vi "Histogram.vi"(0 "image in":refnum<class "MSC Image.lvclass">, 5 "error in (no error)":errorcluster) -> (14 "image out":refnum<class "MSC Image.lvclass">, 15 "R":T1, 16 "G":T1, 17 "B":T1, 19 "error out":errorcluster)   [LabVIEW 2014, in "MSC Image.lvclass"]
doc: "Calculates the histogram of the image. You can wire the outputs directly to a XY Graph.\n\nThe image type double can lead to overflows."
uses:
  MSC Image.lvclass
  <vilib>/Analysis/NI_AALPro.lvlib
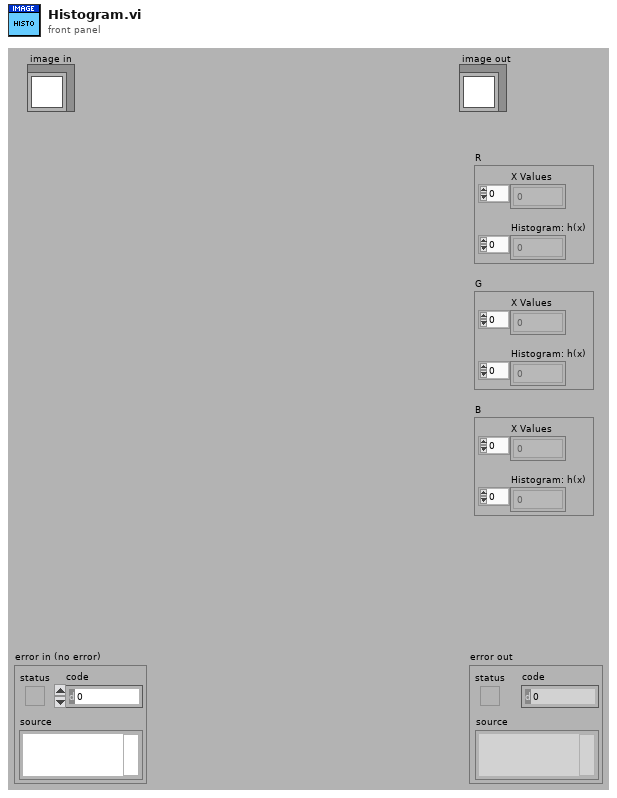
[diagram p1: front panel]
types:
  T1 = cluster{"X Values":dbl[], "Histogram: h(x)":dbl[]}
  T2 = typedef "MSC Image.lvclass/Image Type.ctl" = i32
  T3 = cluster{"X Values":dbl[], "Histogram: h(x)":i32[]}
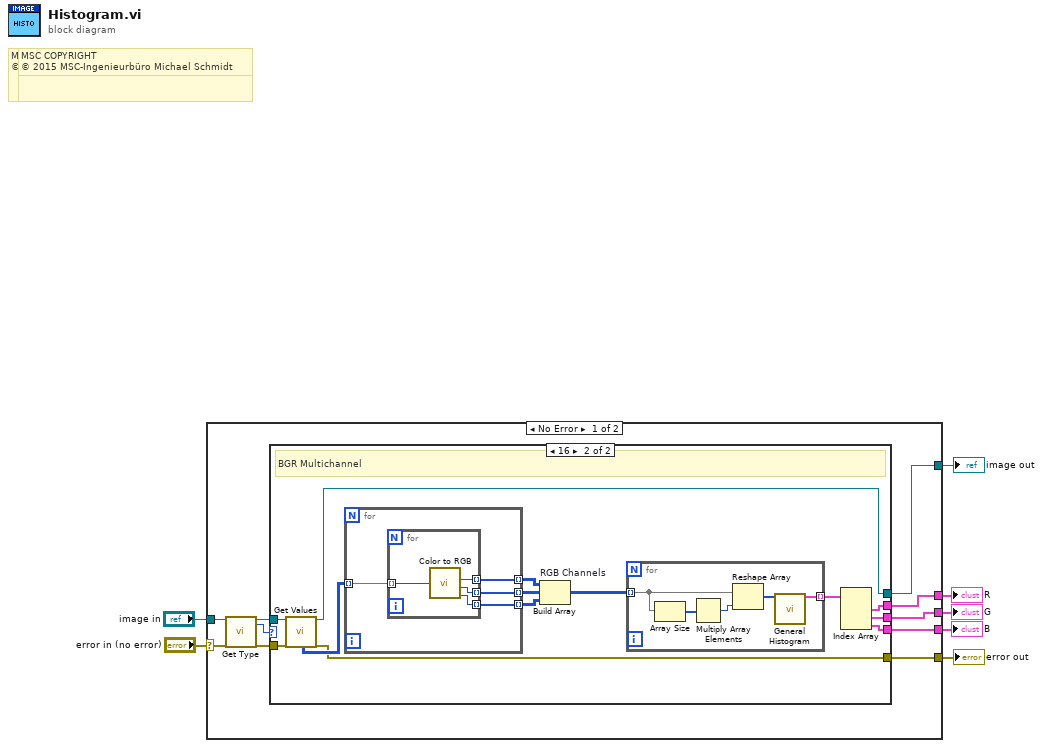
[diagram p0: block diagram]
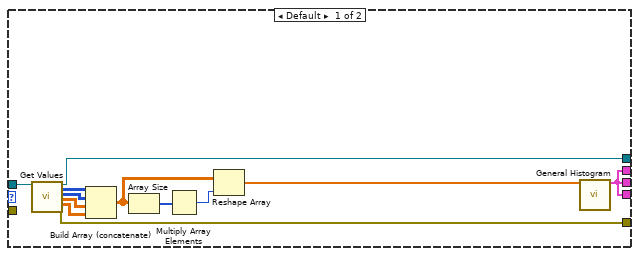
[diagram p2: hidden frame]
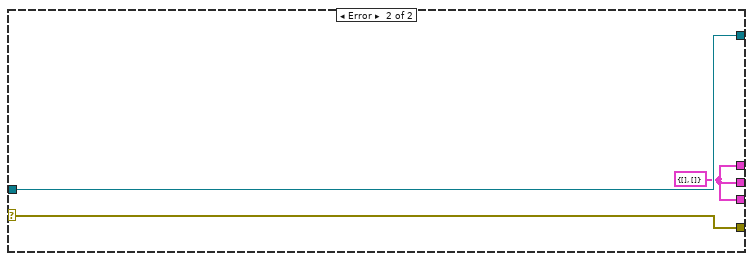
[diagram p3: hidden frame]
diagram:
  # "MSC COPYRIGHT\n© 2016 MSC-Ingenieurbüro Michael Schmidt"
  # "MSC COPYRIGHT\n© 2016 MSC-Ingenieurbüro Michael Schmidt"
  # "MSC COPYRIGHT\n© 2015 MSC-Ingenieurbüro Michael Schmidt"
  # "MSC COPYRIGHT\n© 2015 MSC-Ingenieurbüro Michael Schmidt"
  n1 = case shown="No Error" "error in (no error)" {
    selector: "error in (no error)" -> [w12 w58]
    tunnel: [w13 w58] -> w5
    tunnel: [w17 w57] -> w6
    tunnel: "image in" -> [w10 w57]
    tunnel: [w16 w56] -> w3
    tunnel: [w15 w56] -> w2
    tunnel: [w14 w56] -> w1
    frame No Error {
      n2 = call-dynamic "Get Type.vi"("image in"=w10, "error in (no error)"=w12) -> ("image out"=w9:refnum<class "MSC Image.lvclass">, "Image Type"=w8:T2, "error out"=w11:errorcluster)  [unwired: 15 in]
      n3 = case shown="16" w8 {
        tunnel: w9 -> [w24 w34]
        tunnel: [w23 w32] -> w17
        tunnel: [w29 w37] -> w16
        tunnel: [w29 w36] -> w15
        tunnel: [w29 w35] -> w14
        tunnel: w11 -> [_ w33]
        tunnel: [w18 w30] -> w13
        frame Default {
          n4 = call-dynamic "Get Values.vi"("image in"=w24) -> ("image out"=w23:refnum<class "MSC Image.lvclass">, "imageData U8"=w22:u8[][], "imageData U16"=w21:u16[][], "imageData Single"=w20:sgl[][], "imageData Double"=w19:dbl[][], "error out"=w18:errorcluster)  [unwired: 11 in, 2 out]
          n5 = Build Array (concatenate)(w22, w21, w20, w19) -> (w26:dbl[][])
          n6 = Array Size(array=w26) -> (size(s)=w27:i32[])
          n7 = Multiply Array Elements(1:w27) -> (0:w28:i32)
          n8 = Reshape Array(w26, w28) -> (w25:dbl[])
          n9 = call <vilib>:"General Histogram.vi"("X"=w25) -> ("Histogram Graph"=w29:T3)  [unwired: 10 in, 4 out]
        }
        frame 16 {
          # "BGR Multichannel"
          n10 = call-dynamic "Get Values.vi"("image in"=w34, "error in (no error)"=w33) -> ("imageData BGR"=w31:u32[][], "image out"=w32:refnum<class "MSC Image.lvclass">, "error out"=w30:errorcluster)  [unwired: 10 in, 5 out]
          n11 = for {
            tunnel: w31 -> [w51] mode=indexing
            tunnel: [w50] -> w42 mode=indexing
            tunnel: [w49] -> w41 mode=indexing
            tunnel: [w48] -> w40 mode=indexing
            n12 = for {
              tunnel: w51 -> [w55] mode=indexing
              tunnel: [w54] -> w50 mode=indexing
              tunnel: [w53] -> w49 mode=indexing
              tunnel: [w52] -> w48 mode=indexing
              n13 = call <vilib>:"Color to RGB.vi"("Color"=w55) -> ("R"=w54:u8, "G"=w53:u8, "B"=w52:u8)  [unwired: 1 out]
            }
          }
          n14 = Build Array "RGB Channels"(w42, w41, w40) -> (w39:u8[][][])
          n15 = for {
            tunnel: w39 -> [w45] mode=indexing
            tunnel: [w43] -> w38 mode=indexing
            n16 = Array Size(array=w45) -> (size(s)=w47:i32[])
            n17 = Multiply Array Elements(1:w47) -> (0:w46:i32)
            n18 = Reshape Array(w45, w46) -> (w44:u8[])
            n19 = call <vilib>:"General Histogram.vi"("X"=w44) -> ("Histogram Graph"=w43:T3)  [unwired: 10 in, 4 out]
          }
          n20 = Index Array(array=w38) -> (element #1=w37:T3, element #2=w36:T3, element #3=w35:T3)  [unwired: 3 in]
        }
      }
    }
    frame Error {
      w56 = T3 {"X Values"=[], "Histogram: h(x)"=[]} ("Histogram Graph")
    }
  }
  "error out" <- w5
  "image out" <- w6
  "R" <- w3
  "G" <- w2
  "B" <- w1
